vi "S2DS_Write config file (SubVI).vi"(8 "error in (no error)":errorcluster, 9 "False channel":string[][](array[string]), 10 "All channel parameters":T1 {"Scan parameters"."Y data taking" items=["in both direction", "in up direction only", "in down direction only"]; "Scan parameters"."X data taking" items=["in both direction", "in up direction only", "in down direction only"]}, 11 "file path (use dialog)":path) -> (0 "error out":errorcluster, 3 "file path":path)   [LabVIEW 2025]
uses:
  TYPE DEFS/S2DS_All Channel Parameters.ctl
  TYPE DEFS/S2DS_WC info.ctl
  TYPE DEFS/S2DS_Single WC info.ctl
  TYPE DEFS/S2DS_RC info.ctl
  TYPE DEFS/S2DS_Single RC info.ctl
  TYPE DEFS/S2DS_DAC info new.ctl
  TYPE DEFS/S2DS_Single DC info.ctl
  TYPE DEFS/S2DS_Array Inst Info.ctl
  TYPE DEFS/S2DS_Sweep Info.ctl
  <vilib>/Utility/config.llb/Write Key (String).vi
  <vilib>/Utility/config.llb/NI_LVConfig.lvlib
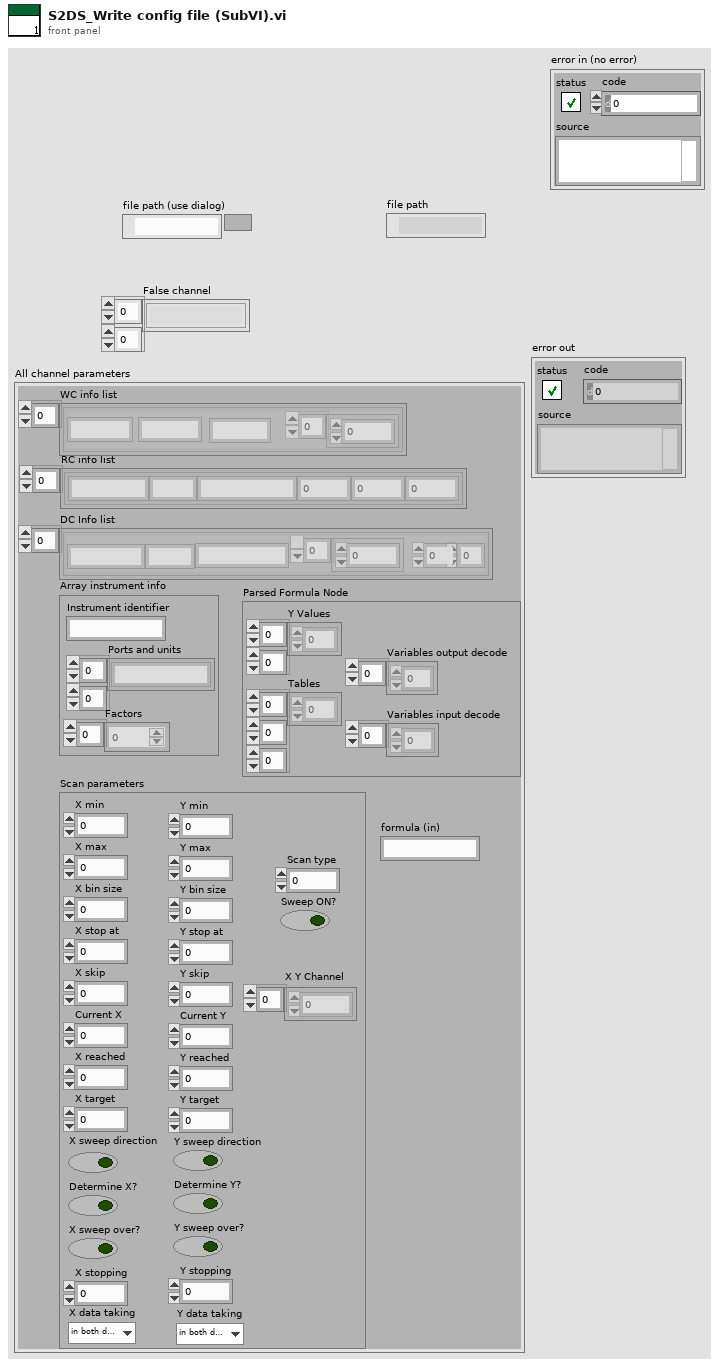
[diagram p1: front panel]
types:
  T1 = typedef "S2DS_All Channel Parameters.ctl" = cluster{"WC info list":T2, "RC info list":T4, "DC Info list":T6, "Array instrument info":T8, "Scan parameters":T9, "Parsed Formula Node":cluster{"Y Values":dbl[][], "Tables":i32[][][], "Variables input decode":i32[], "Variables output decode":i32[]}, "formula (in)":string}
  T2 = typedef "S2DS_WC info.ctl" = T3[]
  T3 = typedef "S2DS_Single WC info.ctl" = cluster{"Instrument identifier":string, "Write channel parameters":dbl[], "Name":string, "Unit":string}
  T4 = typedef "S2DS_RC info.ctl" = T5[]
  T5 = typedef "S2DS_Single RC info.ctl" = cluster{"Instrument identifier":string, "Factor":dbl, "Averaging":i32, "Wait (ms)":i32, "Unit":string, "Name":string}
  T6 = typedef "S2DS_DAC info new.ctl" = T7[]
  T7 = typedef "S2DS_Single DC info.ctl" = cluster{"Operation identifier":string, "DC parameters":dbl[], "U":i32, "V":i32, "Name":string, "Unit":string}
  T8 = typedef "S2DS_Array Inst Info.ctl" = cluster{"Instrument identifier":string, "Ports and units":string[][], "Factors":dbl[]}
  T9 = typedef "S2DS_Sweep Info.ctl" = cluster{"X min":ext, "X max":dbl, "Y min":dbl, "Y max":dbl, "X bin size":dbl, "Y bin size":dbl, "X stop at":dbl, "Y stop at":dbl, "X skip":u64, "Y skip":u64, "Current X":dbl, "Current Y":dbl, "X reached":i32, "Y reached":i32, "X target":dbl, "Y target":dbl, "Sweep ON?":bool, "X sweep direction":bool, "Y sweep direction":bool, "Determine X?":bool, "Determine Y?":bool, "X sweep over?":bool, "Y sweep over?":bool, "Scan type":i32, "X stopping":i32, "Y stopping":i32, "X Y Channel":u16[], "X data taking":u16, "Y data taking":u16}
  T10 = typedef "NI_LVConfig.lvlib/Config Data RefNum.ctl" = refnum<k1>
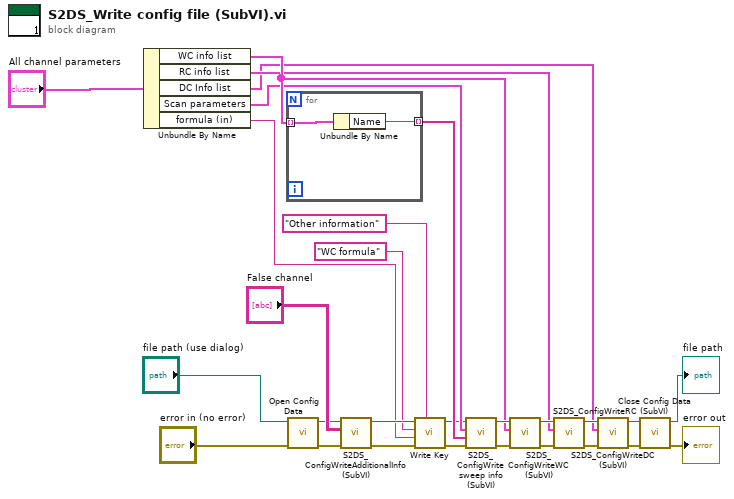
[diagram p0: block diagram]
diagram:
  n1 = Unbundle By Name("All channel parameters") -> ("WC info list"=w12:T2, "RC info list"=w10:T4, "DC Info list"=w9:T6, "Scan parameters"=w8:T9, "formula (in)"=w1:string)
  n2 = for {
    tunnel: w12 -> [w30] mode=indexing
    tunnel: [w29] -> w21 mode=indexing
    n3 = Unbundle By Name(w30) -> ("Name"=w29:string)
  }
  n4 = call <vilib>:"Open Config Data.vi"("error in (no error)"="error in (no error)", "configuration file path"="file path (use dialog)") -> ("error out"=w17:errorcluster, "refnum"=w18:T10)  [unwired: 1 in, 7 out]
  n5 = call "S2DS_ConfigWriteAdditionalInfo (SubVI).vi"("error in (no error)"=w17, "False channel"="False channel", "Refnum in"=w18) -> ("error out"=w4:errorcluster, "Refnum out"=w6:T10)  [unwired: 7 in]
  n6 = call-poly <vilib>:"Write Key.vi"("section"="Other information", "error in (no error)"=w4, "value"=w1, "key"="WC formula" ("section"), "refnum"=w6) -> ("error out"=w3:errorcluster, "refnum out"=w5:T10)  [unwired: 4 in, 1 out]
  n7 = call "S2DS_ConfigWrite sweep info (SubVI).vi"("error in (no error)"=w3, "WC Channel names"=w21, "Scan parameters in"=w8, "Refnum in"=w5) -> ("error out"=w23:errorcluster, "Refnum out"=w22:T10)  [unwired: 6 in]
  n8 = call "S2DS_ConfigWriteWC (SubVI).vi"("error in (no error)"=w23, "WC info list"=w12, "Refnum in"=w22) -> ("error out"=w24:errorcluster, "Refnum out"=w25:T10)  [unwired: 5 in]
  n9 = call "S2DS_ConfigWriteRC (SubVI).vi"("Refnum in"=w25, "RC info list"=w10, "error in"=w24) -> ("Refnum out"=w26:T10, "error out"=w27:errorcluster)  [unwired: 5 in]
  n10 = call "S2DS_ConfigWriteDC (SubVI).vi"("Refnum in"=w26, "DAC info list"=w9, "error in (no error)"=w27) -> ("Refnum out"=w16:T10, "error out"=w15:errorcluster)  [unwired: 4 in]
  n11 = call <vilib>:"Close Config Data.vi"("error in (no error)"=w15, "refnum"=w16) -> ("error out"=→"error out":errorcluster, "file path"=→"file path":path)  [unwired: 1 in, 7 out]
